vi "unix_time_to_labview.vi"(1 "Unix time":i64) -> (0 "LabVIEW time":i64)   [LabVIEW 2010]
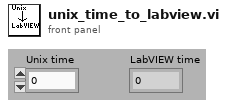
[diagram p1: front panel]
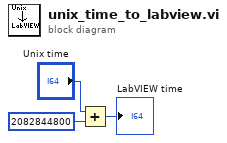
[diagram p0: block diagram]
diagram:
  n1 = Add(x="Unix time", y=i64 2082844800) -> (x+y=→"LabVIEW time":i64)
